vi "filter tags by name.vi"(10 "allowable patterns":string[](array[string]), 11 "tags in":refnum<class "data bus tag description.lvclass">[](array[class])) -> (3 "filtered tags":refnum<class "data bus tag description.lvclass">[](array[class]))   [LabVIEW 2013, in "data bus tag description.lvclass"]
doc: "Filters a list of tags by name, using a pattern match to decide which tags are included or excluded from the filtered list."
uses:
  data bus tag description.lvclass
  data bus tag description.lvclass/data bus tag description.ctl
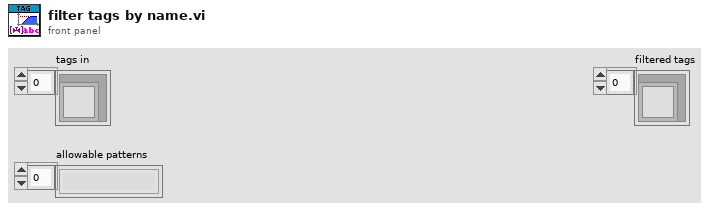
[diagram p1: front panel]
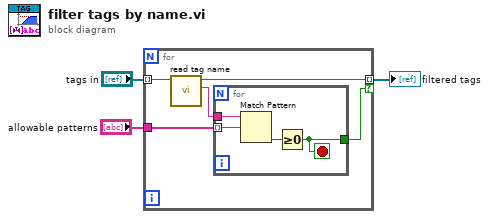
[diagram p0: block diagram]
diagram:
  n1 = for {
    tunnel: [w7] -> w3 mode=indexing if=w4
    tunnel: "tags in" -> [w8] mode=indexing
    tunnel: "allowable patterns" -> [w5]
    n2 = call "read tag name.vi"("system tag in"=w8) -> ("name"=w6:string, "system tag out"=w7:refnum<class "data bus tag description.lvclass">)  [unwired: 8 in, 1 out]
    n3 = for {
      tunnel: w6 -> [w12]
      tunnel: w5 -> [w11] mode=indexing
      tunnel: [w9] -> w4
      stop <- w9 stop-if-true
      n4 = Match Pattern(string=w12, regular expression=w11) -> (offset past match=w10:i32)  [unwired: 1 in, 3 out]
      n5 = Greater Or Equal To 0?(x=w10) -> (x >= 0?=w9:bool)
    }
  }
  "filtered tags" <- w3
